vi "Peak Sound Level.vi"(4 "peak init/cont (init:F)":bool, 6 "weighting filter init/cont (init:F)":bool, 7 "type":enum16{"Type 0", "Type 1"}(ring)=enum."Type 1", 8 "channel info":T2={"sensor sensitivity [mV/EU]"=1000.0, "engineering units"=1, "dB reference [EU]"=1.0, "custom label"="EU", "weighting filter"=0, "pregain [dB]"=0.0} {"pregain [dB]" format="%.2f"; "weighting filter" items=["Linear", "A-weighting", "B-weighting", "C-weighting", "ITU-R 468-4", "Dolby", "CCITT", "C-message"]; "dB reference [EU]" format="%^.1e"; "engineering units" items=["custom..."=0, "V"=1, "A"=21, "Pa"=2, "N"=20, "g"=3, "m/s^2"=4, "m/s"=5, "m"=6, "mm/s"=12, "mm"=13, "microns/s"=14, "microns"=15, "in/s^2"=7, "in/s"=8, "in"=9, "mils/s"=10, "mils"=11, "rad/s^2"=16, "rad/s"=17, "rad"=18, "strain"=19]; "sensor sensitivity [mV/EU]" format="%.2f"}, 9 "weighting filter":T1(ring), 10 "sampling frequency [Hz]":dbl=10000.0 format="%.2f", 11 "scaled signal [EU]":dbl[](array[numeric]) format="%.2f") -> (0 "weighting conflict":bool, 1 "max freq within tolerances [Hz]":dbl format="%.2f", 2 "unit label":string, 3 "peak sound level [dB EU]":dbl format="%.2f")   [LabVIEW 2017]
doc: "Computes the peak sound level of the input signal."
uses:
  <vilib>/addons/Sound and Vibration/compatibility/Controls/svl_Channel Info.ctl
  <vilib>/addons/Sound and Vibration/compatibility/Controls/svl_Engineering Units Text Ring.ctl
  <vilib>/addons/Sound and Vibration/compatibility/Controls/svl_Weighting Filter Text Ring.ctl
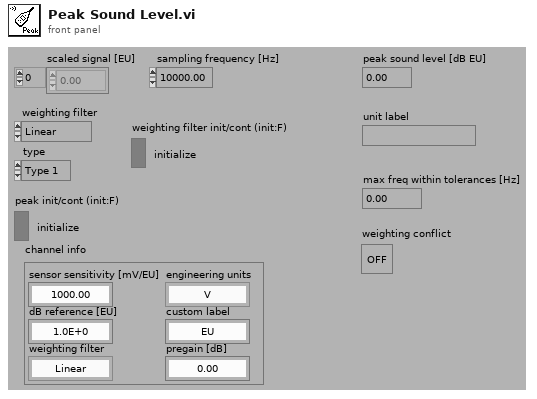
[diagram p1: front panel]
types:
  T1 = enum16{"Linear", "A-weighting", "B-weighting", "C-weighting"}
  T2 = typedef "svl_Channel Info.ctl" = cluster{"sensor sensitivity [mV/EU]":dbl, "engineering units":T3, "dB reference [EU]":dbl, "custom label":string, "weighting filter":T4, "pregain [dB]":dbl}
  T3 = typedef "svl_Engineering Units Text Ring.ctl" = u16
  T4 = typedef "svl_Weighting Filter Text Ring.ctl" = u16
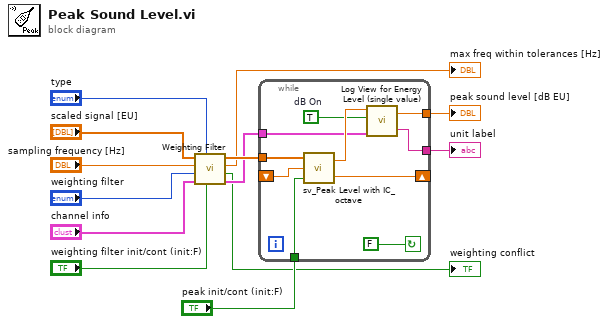
[diagram p0: block diagram]
diagram:
  n1 = call <vilib>:"Weighting Filter.vi"("weighting filter init/cont (init:F)"="weighting filter init/cont (init:F)", "type"="type", "channel info IN"="channel info", "weighting filter"="weighting filter", "sampling frequency [Hz]"="sampling frequency [Hz]", "scaled signal [EU]"="scaled signal [EU]") -> ("channel info OUT"=w4:T2, "weighting conflict"=→"weighting conflict":bool, "max freq within tolerances [Hz]"=→"max freq within tolerances [Hz]":dbl, "weighted signal [EU]"=w9:dbl[])
  n2 = while {
    tunnel: w4 -> [w15]
    tunnel: [w16] -> w11
    tunnel: [w17] -> w12
    tunnel: "peak init/cont (init:F)" -> [w20]
    tunnel: w9 -> [w21]
    shift-left: _ -> [w23]
    shift-right: [w22] -> _
    stop <- FALSE continue-if-true
    w18 = TRUE  # dB On
    n3 = call <vilib>:"sv_Peak Level with IC_octave.vi"("init/cont (init:F)"=w20, "initial peak level"=w23, "scaled signal [EU]"=w21) -> ("final peak level"=w22:dbl, "peak level"=w19:dbl)
    n4 = call <vilib>:"Log View for Energy Level (single value).vi"("channel info"=w15, "dB On (T)"=w18, "energy level [EU^2 rms]"=w19) -> ("unit label"=w16:string, "log view [dB EU]"=w17:dbl)  [unwired: 1 in]
  }
  "peak sound level [dB EU]" <- w12
  "unit label" <- w11
